vi "Read All References.vi"(4 "Error In":errorcluster, 7 "Plugin Names":T1) -> (0 "Error Out":errorcluster, 3 "Reference Out":refnum<vi> caption="VI Refnum")   [LabVIEW 2015, in "Plugin References.lvlib"]
uses:
  Plugin References.lvlib
  _libraries/Startup Processes/_typedefs/Subpanel Names.ctl
  _libraries/Startup Processes/Startup Processes.lvlib
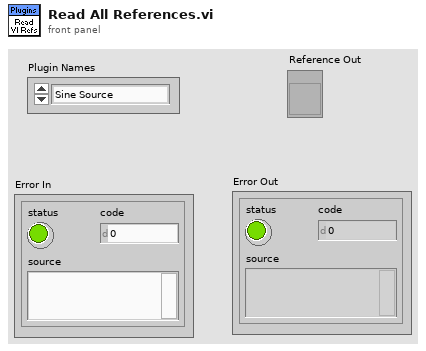
[diagram p1: front panel]
types:
  T1 = typedef "Startup Processes.lvlib/Subpanel Names.ctl" = enum16{"Sine Source", "Ramp Source", "Hen House TC", "Dog House TC", "Out House TC"}
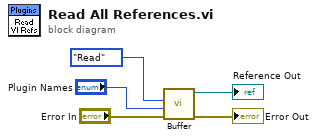
[diagram p0: block diagram]
diagram:
  n1 = call "Buffer.vi"("Error In"="Error In", "Plugin Names"="Plugin Names", "Function"=enum16{"Read", "Insert"}."Read") -> ("Error Out"=→"Error Out":errorcluster, "VI Ref Out"=→"Reference Out":refnum<vi>)  [unwired: 3 in]
